vi "CRYView Init.vi"   [LabVIEW 2013]
uses:
  Control/Graph Main Info Cluster.ctl
  CRYView Global.vi
  CRYMainGlobal.vi
  CRYNew View Global.vi
panel:
  # "View Initialization."
types:
  T1 = typedef "Graph Main Info Cluster.ctl" = cluster{"Selected_BarIdx":i32, "Selected_PanelIdx":i32, "Graph Main VIRef":refnum<vi>, "ToolBarClick":bool, "Spliter Ref Array":refnum<vi>[], "Panel Ref Array":refnum<vi>[], "Spliter_matrix":i32[][], "Panel_matrix":i32[][], "child_spliterIdx_matrix":i32[][], "split_pos_matrix":i32[][], "Title State":bool, "sQueueName":string, "Frame nID":i32, "Graph VIRef Array":cluster{"Graph VIRef":refnum<vi>, "Panel Idx":i32, "Frame VIRef":refnum<vi>, "Icon Ring":i32, "Graph Type":string}[], "View Type":string}
  T2 = cluster{"sAction":string, "sData":string, "nData":i32, "pVIRef":refnum<vi>}[]
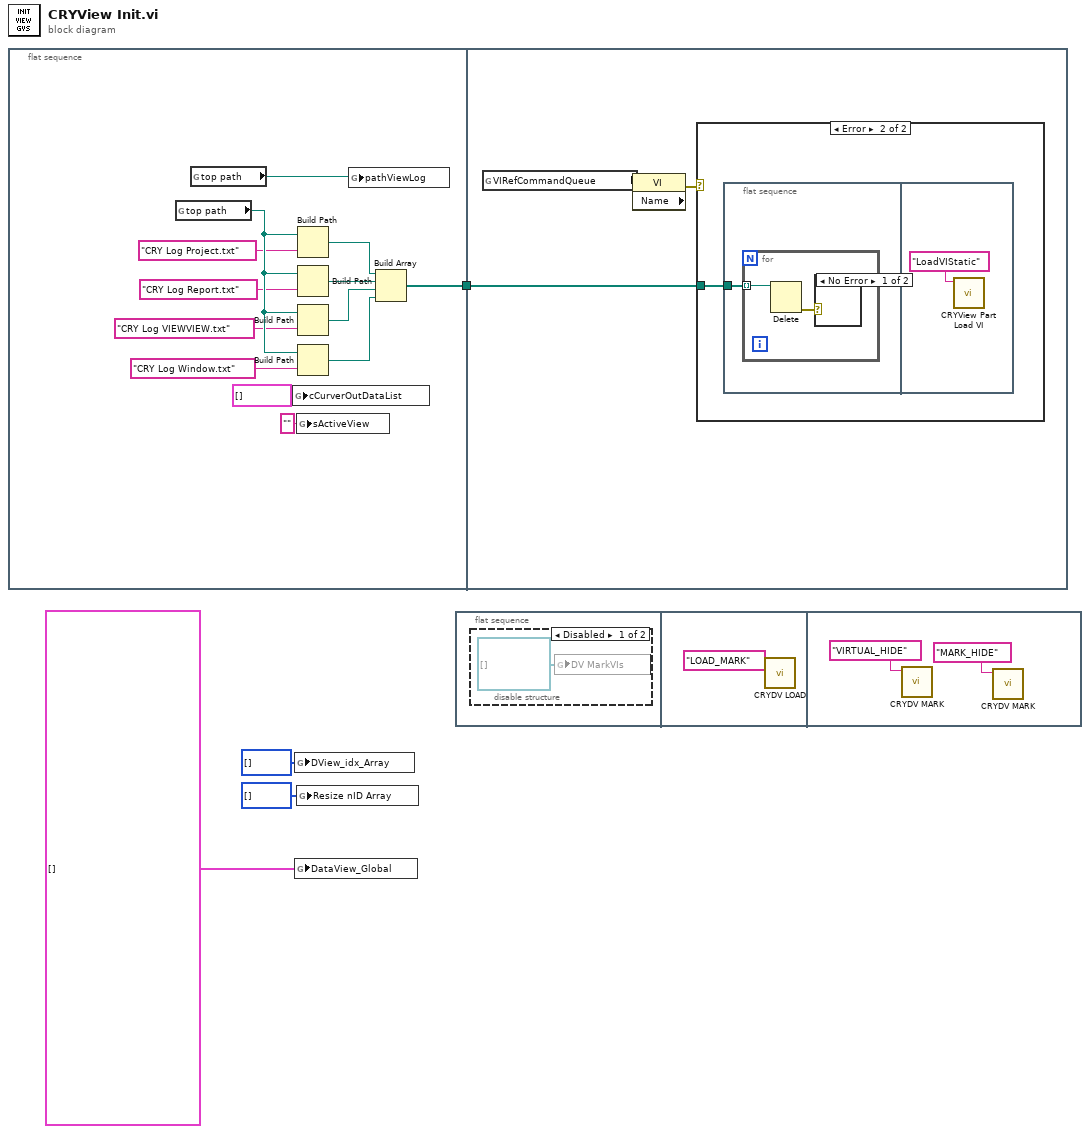
[diagram p0: block diagram]
diagram:
  n1 = flat-sequence {
    tunnel: [w7] -> w4
    tunnel: w4 -> [w19]
    frame #0 {
      n2 = global read "CRYMainGlobal.vi" "top path"() -> (w16:path)
      n3 = global read "CRYMainGlobal.vi" "top path"() -> (w17:path)
      n4 = global write "CRYView Global.vi" "cCurverOutDataList"(T2 [] ("cCurverOutDataList")) -> ()
      n5 = global write "CRYView Global.vi" "sActiveView"("" ("sUseView")) -> ()
      n6 = Build Path(base path=w16, name or relative path="CRY Log Project.txt") -> (appended path=w11:path)
      n7 = Build Path(base path=w16, name or relative path="CRY Log Report.txt") -> (appended path=w10:path)
      n8 = Build Path(base path=w16, name or relative path="CRY Log VIEWVIEW.txt") -> (appended path=w9:path)
      n9 = Build Path(base path=w16, name or relative path="CRY Log Window.txt") -> (appended path=w8:path)
      n10 = global write "CRYView Global.vi" "pathViewLog"(w17) -> ()
      n11 = Build Array(w11, w10, w9, w8) -> (w7:path[])
    }
    frame #1 {
      n12 = global read "CRYView Global.vi" "VIRefCommandQueue"() -> (w18:refnum<vi>)
      n13 = property class="VI" props=["Name"](reference=w18) -> (error out=w20:errorcluster)  [unwired: 1 in, 2 out]
      n14 = case shown="Error" w20 {
        tunnel: w19 -> [_ w21]
        frame No Error {
        }
        frame Error {
          n15 = flat-sequence {
            tunnel: w21 -> [w22]
            frame #0 {
              n16 = for {
                tunnel: w22 -> [w24] mode=indexing
                n17 = Delete(path (use dialog)=w24) -> (error out=w23:errorcluster)  [unwired: 4 in, 2 out]
                n18 = case shown="No Error" w23 {
                  frame No Error {
                  }
                  frame Error {
                  }
                }
              }
            }
            frame #1 {
              n19 = call "CRYView Part Load VI.vi"("sAction"="LoadVIStatic") -> ()  [unwired: 10 in, 1 out]
            }
          }
        }
      }
    }
  }
  n20 = global write "CRYNew View Global.vi" "DView_idx_Array"(i32[] [] ("DView_idx_Array")) -> ()
  n21 = global write "CRYNew View Global.vi" "DataView_Global"(T1[] [] ("DataView_Global")) -> ()
  n22 = global write "CRYNew View Global.vi" "Resize nID Array"(i32[] [] ("Resize nID Array")) -> ()
  n23 = flat-sequence {
    frame #0 {
      n24 = disable-structure shown="Disabled" {
        frame Disabled {
          n25 = global write "CRYNew View Global.vi" "DV MarkVIs"(refnum<vi>[] [] ("DV MarkVIs")) -> ()
        }
        frame Enabled {
        }
      }
    }
    frame #1 {
      n26 = call "CRYDV LOAD.vi"("sAction"="LOAD_MARK") -> ()  [unwired: 7 in, 4 out]
    }
    frame #2 {
      n27 = call "CRYDV MARK.vi"("sAction"="VIRTUAL_HIDE") -> ()  [unwired: 9 in, 1 out]
      n28 = call "CRYDV MARK.vi"("sAction"="MARK_HIDE") -> ()  [unwired: 9 in, 1 out]
    }
  }
